vi "Camera continuous acquisition.vi"() -> ()   [LabVIEW 2016]
uses:
  Classes/Controller/Camera/Camera Folder/Machine Vision.ctl
  Classes/Controller/Camera/Camera Folder/Camera.lvclass
panel:
  in  "Stop":bool
  out "Image 3":T1(plugin-control)
  out "Camera 2":dbl[](array[numeric])=[0.23163148760795593, 0.18427667021751404] format="%#_8g"
  in  "Machine Vision":T2=enum."tpcb_hole"
  out "Numeric":dbl
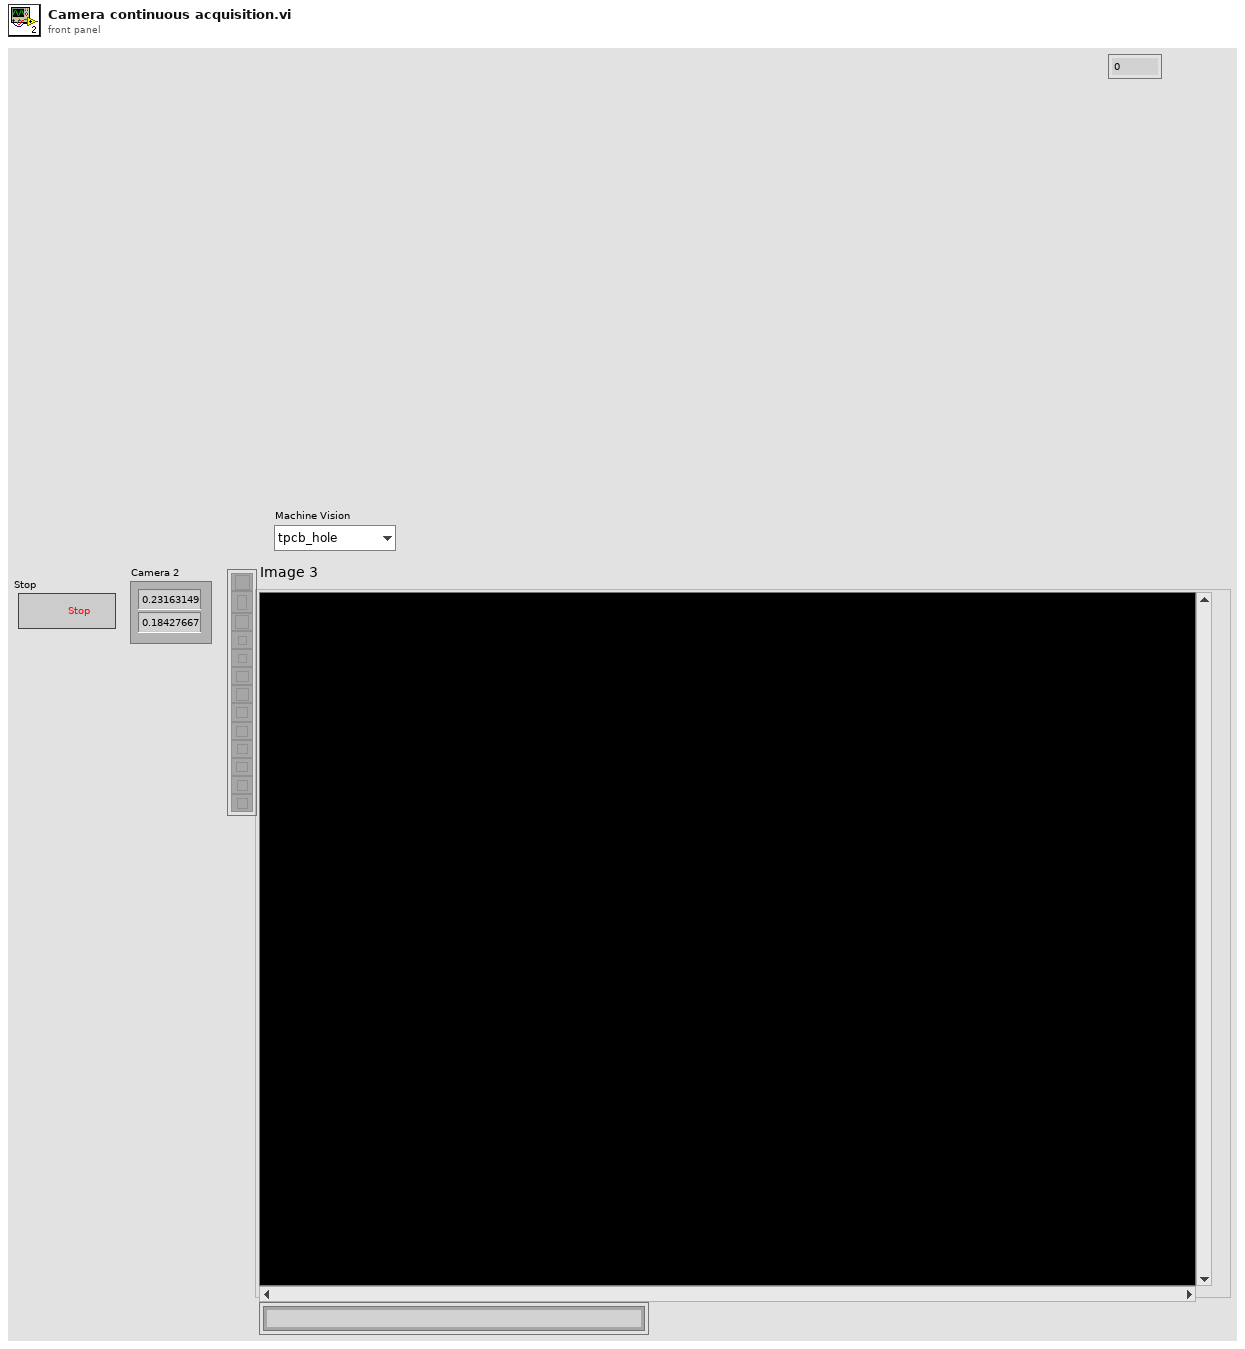
[diagram p1: front panel]
types:
  T1 = typedef "IMAQ Image.ctl" = refnum<image>
  T2 = typedef "Camera.lvclass/Machine Vision.ctl" = enum16{"top left corner", "top right corner", "bottom left corner", "bottom right corner", "bottom left chip", "top right chip", "None", "tracker fiducial", "chip cross 2", "chip cross", "Focus", "INTT HDI Mark", "INTT Sensor Cross", "INTT Chip Corner", "HPK Silicon", "Circle", "tpcb_hole"}
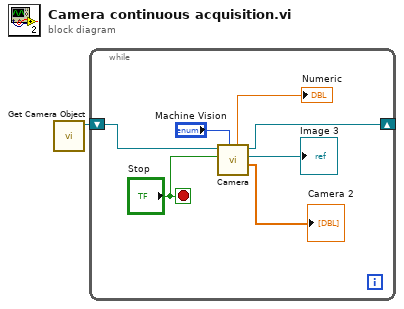
[diagram p0: block diagram]
diagram:
  n1 = call "Get Camera Object.vi"() -> ("Camera out"=w1:refnum<class "Camera.lvclass">)  [unwired: 10 in, 1 out]
  n2 = while {
    shift-right: [w7] -> _
    shift-left: w1 -> [w8]
    stop <- "Stop" stop-if-true
    n3 = call "Camera.vi"("Machine Vision"="Machine Vision", "Stop"="Stop", "Camera in"=w8) -> ("Camera"=→"Camera 2":dbl[], "Image"=→"Image 3":T1, "Camera out"=w7:refnum<class "Camera.lvclass">, "Focus output"=→"Numeric":dbl)  [unwired: 4 in, 1 out]
  }
